vi "create_ch_file.vi"(4 "device factory id":string, 5 "mouse id":string, 6 "device name":string, 7 "channel name":string, 8 "error in (no error)":errorcluster, 9 "sampling rate":dbl, 10 "time stamp":timestamp, 11 "appended path":path) -> (0 "error out":errorcluster, 3 "refnum out":refnum<file>)   [LabVIEW 2017]
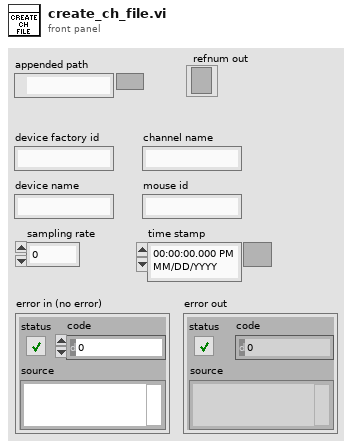
[diagram p1: front panel]
types:
  T1 = enum16{"open", "replace", "create", "open or create", "replace or create", "replace or create with confirmation"}
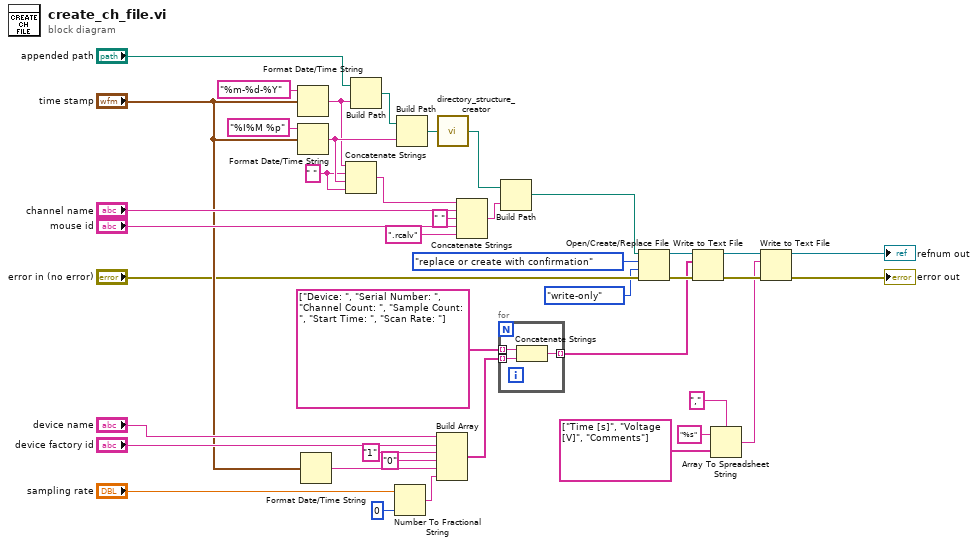
[diagram p0: block diagram]
diagram:
  w36 = " " ("string")
  n1 = Format Date/Time String(time format string (%c)="%m-%d-%Y", seconds (now)="time stamp") -> (date/time string=w35:string)  [unwired: 1 in]
  n2 = Format Date/Time String(time format string (%c)="%I%M %p", seconds (now)="time stamp") -> (date/time string=w37:string)  [unwired: 1 in]
  n3 = Format Date/Time String(seconds (now)="time stamp") -> (date/time string=w24:string)  [unwired: 2 in]
  n4 = Concatenate Strings(w35, w36, w37, w36) -> (w41:string)
  n5 = Build Path(base path="appended path", name or relative path=w35) -> (appended path=w31:path)
  n6 = Number To Fractional String(number="sampling rate", precision (6)=i16 0) -> (F-format string=w25:string)  [unwired: 2 in]
  n7 = Build Path(base path=w31, name or relative path=w37) -> (appended path=w32:path)
  n8 = Build Array("device name", "device factory id", "1" ("element"), "0" ("element"), w24, w25) -> (w29:string[])
  n9 = call "directory_structure_creator.vi"("Path to be created"=w32) -> ("Duplicate \"Path to be created\""=w39:path)
  n10 = Concatenate Strings(w41, "channel name", " " ("string"), "mouse id", ".rcalv" ("string")) -> (w40:string)
  n11 = for {
    tunnel: string[] ["Device: ", "Serial Number: ", "Channel Count: ", "Sample Count: ", "Start Time: ", "Scan Rate: "] -> [w44] mode=indexing
    tunnel: w29 -> [w43] mode=indexing
    tunnel: [w42] -> w11 mode=indexing
    n12 = Concatenate Strings(w44, w43) -> (w42:string)
  }
  n13 = Build Path(base path=w39, name or relative path=w40) -> (appended path=w15:path)
  n14 = Open/Create/Replace File(file path (use dialog)=w15, error in="error in (no error)", operation (0:open)=T1."replace or create with confirmation", access (0:read/write)=enum16{"read/write", "read-only", "write-only"}."write-only") -> (refnum out=w12:refnum<file>, error out=w13:errorcluster)  [unwired: 2 in, 1 out]
  n15 = Write to Text File(file (use dialog)=w12, text=w11, error in=w13) -> (refnum out=w9:refnum<file>, error out=w10:errorcluster)  [unwired: 1 in, 1 out]
  n16 = Array To Spreadsheet String(delimiter (Tab)=",", array=string[] ["Time [s]", "Voltage [V]", "Comments"], 3:"%s" ("format string")) -> (spreadsheet string=w3:string)
  n17 = Write to Text File(file (use dialog)=w9, text=w3, error in=w10) -> (refnum out=→"refnum out":refnum<file>, error out=→"error out":errorcluster)  [unwired: 1 in, 1 out]
